vi "Get DG by Index.vi"(8 "error in (no error)":errorcluster, 10 "index":i32=1 min=1, 11 "BME_DG_System in":refnum<class "BME_DG_System.lvclass">) -> (0 "error out":errorcluster, 2 "BME_DG_Base.lvclass":refnum<class "BME_DG_Base.lvclass">, 3 "BME_DG_System out":refnum<class "BME_DG_System.lvclass">)   [LabVIEW 2009, in "POLARIS BME DG.lvlib" / "BME_DG_System.lvclass"]
uses:
  BME_DG_System.lvclass
  BME_DG_Base/BME_DG_Base.lvclass
  BME_DG_System.lvclass/BME_DG_System.ctl
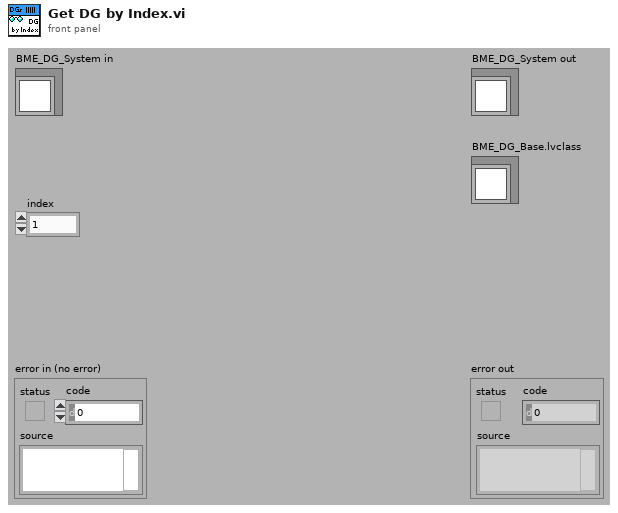
[diagram p1: front panel]
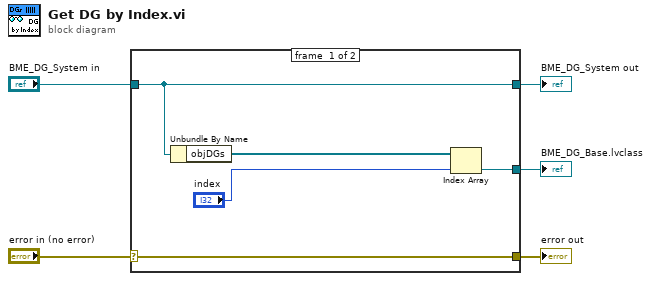
[diagram p0: block diagram]
diagram:
  n1 = case shown="No Error" "error in (no error)" {
    selector: "error in (no error)" -> [w10 w11]
    tunnel: [w10 w11] -> w4
    tunnel: [w9 w12] -> w2
    tunnel: "BME_DG_System in" -> [w9 w12]
    tunnel: [w6 _] -> w1
    frame #0 {
      n2 = Unbundle By Name(w9) -> ("objDGs"=w8:refnum<class "BME_DG_Base.lvclass">[])
      n3 = Index Array(array=w8, index="index") -> (element=w6:refnum<class "BME_DG_Base.lvclass">)
    }
    frame #1 {
    }
  }
  "error out" <- w4
  "BME_DG_System out" <- w2
  "BME_DG_Base.lvclass" <- w1
